vi "db readonly.vi"(8 "error in (no error)":errorcluster, 10 "zDbName":string, 11 "db":dbl) -> (0 "error out":errorcluster, 2 "function return":i32, 3 "db out":dbl)   [LabVIEW 2020, in "sqlite3.lvlib"]
uses:
  sqlite3.lvlib
  errstr.vi
  bin/sqlite3_64.dll
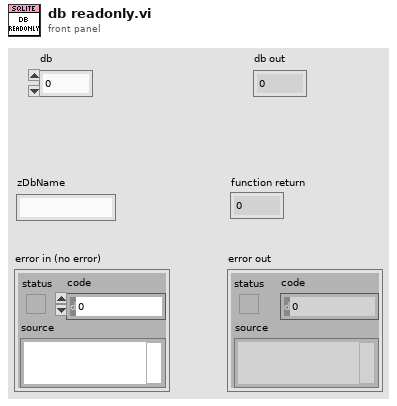
[diagram p1: front panel]
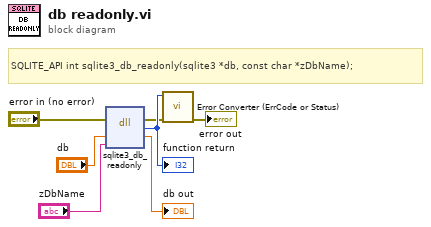
[diagram p0: block diagram]
diagram:
  # "SQLITE_API int sqlite3_db_readonly(sqlite3 *db, const char *zDbName);"
  n1 = dll-call lib="C:/Users/Fred.Guo/Desktop/Database-configuration/externals/sqlite3/Source/bin/sqlite3_*.*" fn="sqlite3_db_readonly"(error in="error in (no error)", "db"="db", "zDbName"="zDbName") -> (error out=w2:errorcluster, w7:i32, "db"=→"db out":dbl)  [unwired: 3 in, 1 out]
  "function return" <- w7
  n2 = call "Error Converter (ErrCode or Status).vi"("error in (no error)"=w2, "error code"=w7) -> ("error out"=→"error out":errorcluster)  [unwired: 9 in]
